vi "Vision Processing.vi"(4 "error in (no error)":errorcluster, 7 "Image Size":T1=enum."320x240") -> ()   [LabVIEW 2015]
doc: "This VI runs in parallel to other tasks. It gets images from the camera, processes them for color or shape and uses commands or globals to affect the behavior of other subsystems."
uses:
  <vilib>/Rock Robotics/WPI/Camera/WPI_CameraImageSize.ctl
  Labview/2016 Vision Tracking/Vision Support Code/Camera Types.ctl
  <vilib>/Rock Robotics/WPI/Camera/WPI_CameraWhite Balance Values.ctl
  <vilib>/Rock Robotics/WPI/Camera/WPI_CameraExposure Values.ctl
  <vilib>/Rock Robotics/WPI/Camera/WPI_CameraFrameRate.ctl
  Framework/Robot Global Data.vi
  <vilib>/vision/NI_Vision_Development_Module.lvlib
panel:
  in  "Max Limit %":dbl=0.12 format="%#_13g"
  in  "Min Limit %":dbl=0.12 format="%#_13g"
  in  "Image Size 2":T1=enum."320x240"
  out "ms to process 2":u32
  in  "error in (no error) 2":errorcluster
  out "ms to process":u32
  in  "LED Color":T2={"Hue"={23.67058792990901, 48.923317529462665}, "Sat"={66.78571428571429, 255.0}, "Val"={48.571428571428584, 255.0}} {"Hue" scale=0.0..255.0 scale format="%#_3g"}
  out "Qualified Particles":i32
  in  "Score Threshold":dbl=75.0
  in  "Aspect Fudge Factor":dbl=1.0
  in  "Min Score Threshold":i32=75
  in  "Camera Type":T3=enum."MS HD3000 square"
  in  "Emphasize Limit Tests":bool=TRUE
  out "Masked 2":T4(plugin-control)
  in  "Display Mask":bool=TRUE
  out "Original Image":T4(plugin-control)
  in  "Display Original":bool=TRUE
  out "Sorted Particle Scores":T5(array[cluster]) {"Moment Factor" format="%#_3g"; "Aspect Ratio" format="%#_3g"; "Area to CH" format="%#_3g"; "X" format="%#_3g"; "Y" format="%#_3g"}
  out "Highest Avg Score":dbl
  out "Detected Targets":T6(array[cluster]) {"Normalized Rect"."Numeric 5" format="%#_2g"; "Normalized Rect"."Numeric 3" format="%#_2g"; "Normalized Rect"."Numeric 2" format="%#_2g"; "Normalized Rect"."Numeric" format="%#_2g"}
  out "fps":dbl
  out "Masked":T4(plugin-control)
  # "Density Profile"
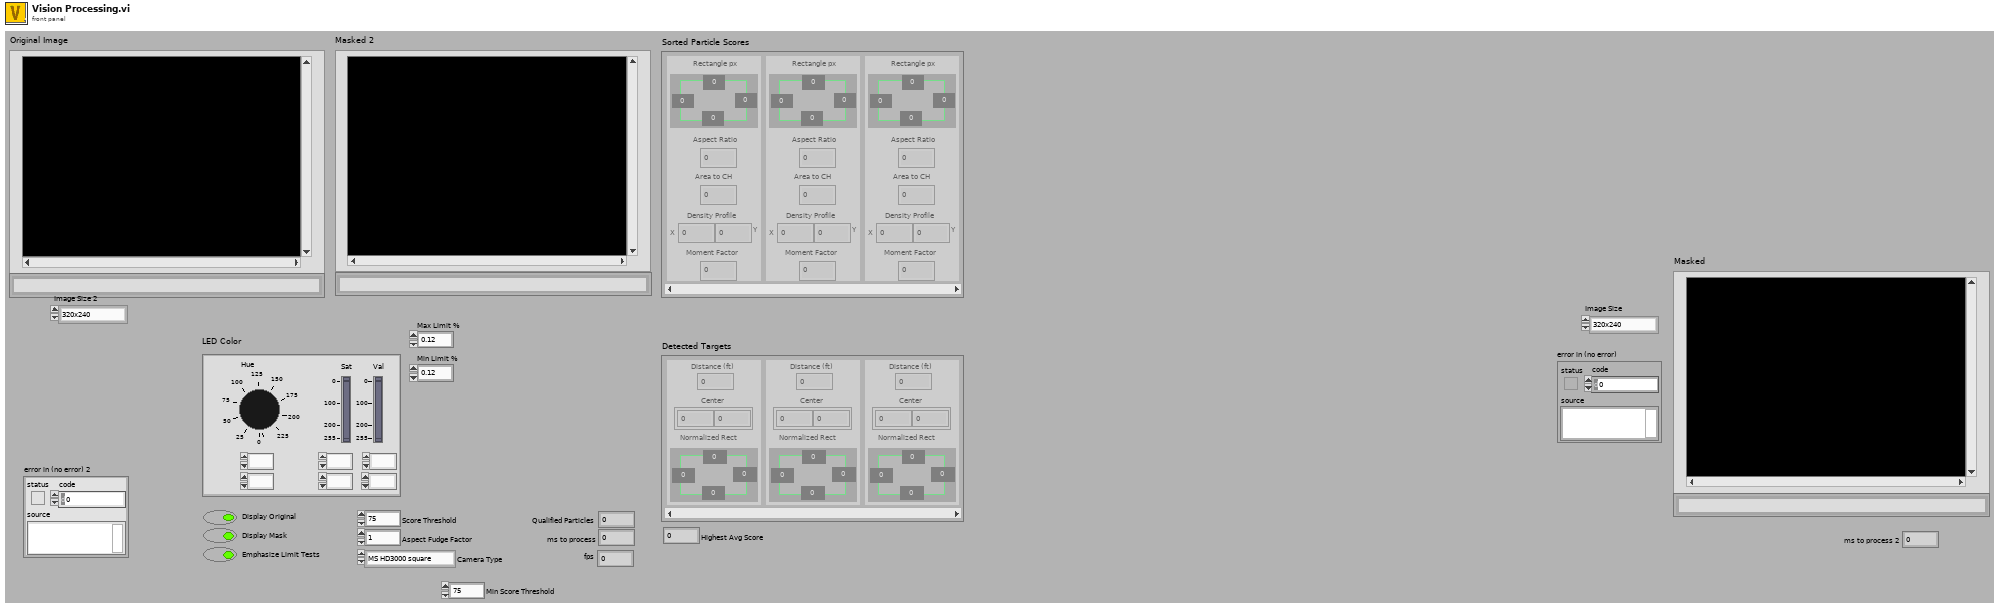
[diagram p1: front panel]
types:
  T1 = typedef "WPI_CameraImageSize.ctl" = enum16{"640x480", "320x240", "160x120", "Custom"}
  T2 = cluster{"Hue":cluster{dbl, dbl}, "Sat":cluster{dbl, dbl}, "Val":cluster{dbl, dbl}}
  T3 = typedef "Camera Types.ctl" = enum16{"206", "1011", "1013", "MS HD3000 square", "MS HD3000 640x480"}
  T4 = typedef "IMAQ Image.ctl" = refnum<image>
  T5 = cluster{"Rectangle px":cluster{"Numeric":dbl, "Numeric 2":dbl, "Numeric 3":dbl, "Numeric 5":dbl}, "Aspect Ratio":dbl, "Area to CH":dbl, "X":dbl, "Y":dbl, "Moment Factor":dbl}[]
  T6 = cluster{"Distance (ft)":dbl, "Center":cluster{dbl, dbl}, "Normalized Rect":cluster{"Numeric":dbl, "Numeric 2":dbl, "Numeric 3":dbl, "Numeric 5":dbl}}[]
  T7 = typedef "WPI_CameraFrameRate.ctl" = u32
  T8 = typedef "WPI_CameraExposure Values.ctl" = enum16{"Auto", "Flicker-free 50 Hz", "Flicker-free 60 Hz", "Hold current", "Custom"}
  T9 = typedef "WPI_CameraWhite Balance Values.ctl" = enum16{"Auto", "Fixed indoor", "Fixed outdoor 1", "Fixed outdoor 2", "Fixed fluorescent 1", "Fixed fluorescent 2", "Hold current", "Custom"}
  T10 = typedef "Image Type" = u32
  T11 = typedef "Particle Parameters" = i32
  T12 = typedef "WPI_CameraDevRef.ctl" = cluster{"Camera Address":string, "CameraStatus":errorcluster}
  T13 = cluster{"Bounding box":cluster{"left":dbl, "top":dbl, "right":dbl, "bottom":dbl}, "Aspect Ratio":dbl, "Area to CH":dbl, "X Mask":dbl, "Y Mask":dbl, "Moment":dbl}[]
  T14 = cluster{"Rectangle":cluster{"Numeric":dbl, "Numeric 2":dbl, "Numeric 3":dbl, "Numeric 5":dbl}, "L":dbl, "Area to CH":dbl, "X":dbl, "Y":dbl, "Moment Factor":dbl}[]
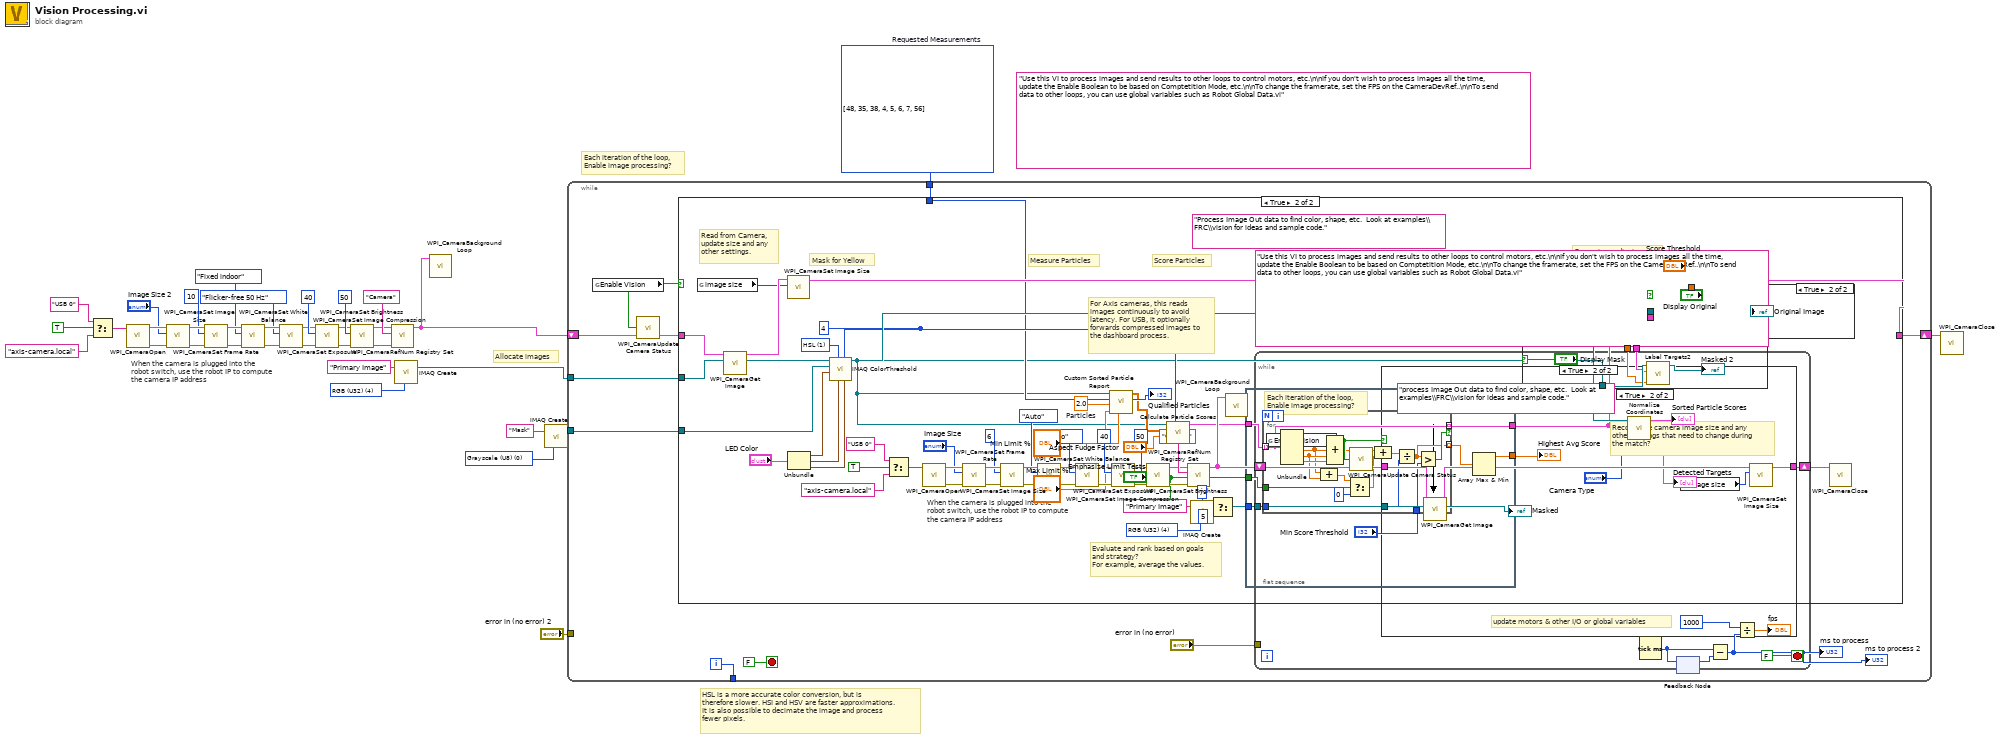
[diagram p0: block diagram]
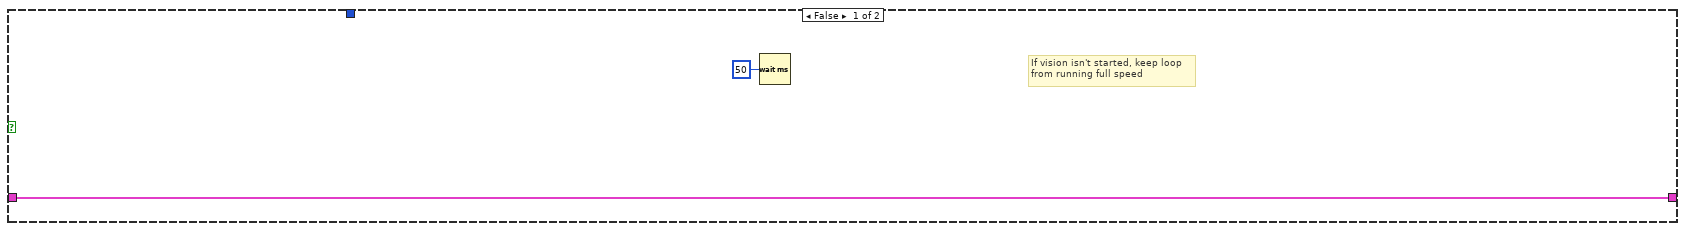
[diagram p2: hidden frame]
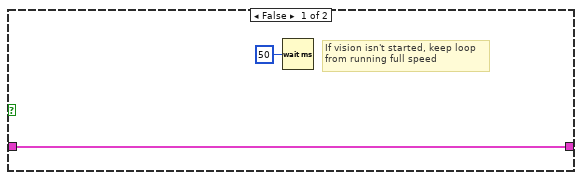
[diagram p5: hidden frame]
diagram:
  w29 = T10 4 items=["Grayscale (U8)", "Grayscale (I16)", "Grayscale (SGL)", "Complex (CSG)", "RGB (U32)", "HSL (U32)", "RGB (U64)"] ("Image Type")
  (unwired) "Use this VI to process images and send results to other loops to control motors, etc.\n\nIf you don't wish to process images all the time, update the Enable Boolean to be based on Comptetition Mode, etc.\n\nTo change the framerate, set the FPS on the CameraDevRef..\n\nTo send data to other loops, you can use global variables such as Robot Global Data.vi"
  w32 = T11[] [48, 35, 38, 4, 5, 6, 7, 56] items=["Center of Mass X", "Center of Mass Y", "First Pixel X", "First Pixel Y", "Bounding Rect Left", "Bounding Rect Top", "Bounding Rect Right", "Bounding Rect Bottom", "Max Feret Diameter Start X", "Max Feret Diameter Start Y", "Max Feret Diameter End X", "Max Feret Diameter End Y", "Max Horiz. Segment Length Left", "Max Horiz. Segment Length Right", "Max Horiz. Segment Length Row", "-", "Bounding Rect Width", "Bounding Rect Height", "Bounding Rect Diagonal", "Perimeter", "Convex Hull Perimeter", "Holes' Perimeter", "Max Feret Diameter", "Equivalent Ellipse Major Axis", "Equivalent Ellipse Minor Axis", "Equivalent Ellipse Minor Axis (Feret)", "Equivalent Rect Long Side", "Equivalent Rect Short Side", "Equivalent Rect Diagonal", "Equivalent Rect Short Side (Feret)", "Average Horiz. Segment Length", "Average Vert. Segment Length", "Hydraulic Radius", "Waddel Disk Diameter", "-", "Area", "Holes' Area", "Particle & Holes' Area", "Convex Hull Area", "Image Area", "-", "Number of Holes", "Number of Horiz. Segments", "Number of Vert. Segments", "-", "Orientation", "Max Feret Diameter Orientation", "-", "% Area/Image Area", "% Area/(Particle & Holes' Area)", "Ratio of Equivalent Ellipse Axes", "Ratio of Equivalent Rect Sides", "-", "Elongation Factor", "Compactness Factor", "Heywood Circularity Factor", "Type Factor", "-", "Sum X", "Sum Y", "Sum XX", "Sum XY", "Sum YY", "Sum XXX", "Sum XXY", "Sum XYY", "Sum YYY", "-", "Moment of Inertia XX", "Moment of Inertia XY", "Moment of Inertia YY", "Moment of Inertia XXX", "Moment of Inertia XXY", "Moment of Inertia XYY", "Moment of Inertia YYY", "Norm. Moment of Inertia XX", "Norm. Moment of Inertia XY", "Norm. Moment of Inertia YY", "Norm. Moment of Inertia XXX", "Norm. Moment of Inertia XXY", "Norm. Moment of Inertia XYY", "Norm. Moment of Inertia YYY", "Hu Moment 1", "Hu Moment 2", "Hu Moment 3", "Hu Moment 4", "Hu Moment 5", "Hu Moment 6", "Hu Moment 7"]  # Requested Measurements
  w35 = T10 0 items=["Grayscale (U8)", "Grayscale (I16)", "Grayscale (SGL)", "Complex (CSG)", "RGB (U32)", "HSL (U32)", "RGB (U64)", "Grayscale (U16)"] ("Image Type")
  (unwired) "Use this VI to process images and send results to other loops to control motors, etc.\n\nIf you don't wish to process images all the time, update the Enable Boolean to be based on Comptetition Mode, etc.\n\nTo change the framerate, set the FPS on the CameraDevRef..\n\nTo send data to other loops, you can use global variables such as Robot Global Data.vi"
  w66 = T10 4 items=["Grayscale (U8)", "Grayscale (I16)", "Grayscale (SGL)", "Complex (CSG)", "RGB (U32)", "HSL (U32)", "RGB (U64)"] ("Image Type")
  # "When the camera is plugged into the\nrobot switch, use the robot IP to compute\nthe camera IP address"
  # "Each iteration of the loop,\nEnable image processing?"
  # "HSL is a more accurate color conversion, but is\ntherefore slower. HSI and HSV are faster approximations.\nIt is also possible to decimate the image and process\nfewer pixels."
  # "Allocate images"
  # "When the camera is plugged into the\nrobot switch, use the robot IP to compute\nthe camera IP address"
  # "For Axis cameras, this reads\nimages continuously to avoid\nlatency. For USB, it optionally\nforwards compressed images to\nthe dashboard process."
  n1 = Select(t="USB 0" ("format string"), s=TRUE ("dot notation? (F)"), f="axis-camera.local" ("format string")) -> (s? t:f=w4:string)
  n2 = call <vilib>:"WPI_CameraOpen.vi"("Camera Address"=w4) -> ("error out"=w18:errorcluster, "CameraDevRef"=w19:T12)  [unwired: 1 in, 8 out]
  n3 = call <vilib>:"WPI_CameraSet Image Size.vi"("error in (no error)"=w18, "Image Size"="Image Size 2", "CameraDevRef"=w19) -> ("error out"=w17:errorcluster, "CameraDevRef Out"=w20:T12)  [unwired: 1 in, 6 out]
  n4 = call <vilib>:"WPI_CameraSet Frame Rate.vi"("error in (no error)"=w17, "Frame Rate (fps)"=T7 10, "CameraDevRef"=w20) -> ("error out"=w16:errorcluster, "CameraDevRef Out"=w22:T12)  [unwired: 7 out]
  n5 = call <vilib>:"WPI_CameraSet White Balance.vi"("error in (no error)"=w16, "White Balance"=WPI_CameraWhite_Balance_Values."Fixed indoor", "CameraDevRef"=w22) -> ("error out"=w15:errorcluster, "CameraDevRef Out"=w21:T12)  [unwired: 1 in, 6 out]
  n6 = call <vilib>:"WPI_CameraSet Exposure.vi"("error in (no error)"=w15, "Exposure"=WPI_CameraExposure_Values."Flicker-free 50 Hz", "CameraDevRef"=w21) -> ("error out"=w14:errorcluster, "CameraDevRef Out"=w24:T12)  [unwired: 1 in, 6 out]
  n7 = call <vilib>:"WPI_CameraSet Image Compression.vi"("error in (no error)"=w14, "Compression"=40, "CameraDevRef"=w24) -> ("error out"=w13:errorcluster, "CameraDevRef Out"=w23:T12)  [unwired: 7 out]
  n8 = call <vilib>:"WPI_CameraSet Brightness.vi"("error in (no error)"=w13, "Brightness"=50, "CameraDevRef"=w23) -> ("error out"=w11:errorcluster, "CameraDevRef Out"=w12:T12)  [unwired: 7 out]
  n9 = call <vilib>:"WPI_CameraRefNum Registry Set.vi"("error in (no error)"=w11, "refnum name"="Camera", "CameraDevRef"=w12) -> ("CameraDevRef"=w2:T12)  [unwired: 1 in, 7 out]
  n10 = call "IMAQ Create"("Image Name"="Primary Image", "Image Type"=w29) -> ("New Image"=w1:T4)  [unwired: 2 in, 2 out]
  n11 = call <vilib>:"WPI_CameraBackground Loop.vi"("CameraDevRef"=w2) -> ()  [unwired: 11 in]
  n12 = call "IMAQ Create"("Image Name"="Mask", "Image Type"=w35) -> ("New Image"=w33:T4)  [unwired: 2 in, 2 out]
  n13 = while {
    tunnel: w1 -> [w75]
    tunnel: w33 -> [w79]
    tunnel: w32 -> [w78]
    tunnel: "error in (no error) 2" -> [_]
    tunnel: [w74] -> _
    shift-right: [w71] -> w30
    shift-left: w2 -> [w67]
    i -> [w74]
    stop <- FALSE stop-if-true
    n14 = global read "Robot Global Data.vi" "Enable Vision"() -> (w73:bool)
    n15 = call <vilib>:"WPI_CameraUpdate Camera Status.vi"("CameraDevRef In"=w67, "Enable Vision"=w73) -> ("CameraDevRef Out"=w72:T12)  [unwired: 3 in]
    n16 = case shown="True" w73 {
      tunnel: w79 -> [_ w116]
      tunnel: w78 -> [_ w87]
      tunnel: w72 -> [w81 w111]
      tunnel: w75 -> [_ w110]
      tunnel: [w81 w108] -> w71
      frame False {
        # "If vision isn't started, keep loop\nfrom running full speed"
        n17 = Wait (ms)(milliseconds to wait=u32 50) -> ()  [unwired: 1 out]
      }
      frame True {
        w95 = 4 ("Replace Value")
        w105 = u16 1 items=["RGB", "HSL", "HSV", "HSI"] ("Color Mode")
        (unwired) "Process Image Out data to find color, shape, etc.  Look at examples\\FRC\\vision for ideas and sample code."
        w85 = 2.0  # Particles
        # "Evaluate and rank based on goals\nand strategy?\nFor example, average the values."
        # "Read from Camera,\nupdate size and any\nother settings."
        # "Measure Particles"
        # "Convert coordinates,\ncalculate distance, etc."
        # "Annotation"
        # "Score Particles"
        # "Mask for Yellow"
        n18 = global read "Robot Global Data.vi" "image size"() -> (w92:T1)
        n19 = call <vilib>:"WPI_CameraGet Image.vi"("Image"=w110, "CameraDevRef"=w111) -> ("Image Out"=w96:T4, "CameraDevRef Out"=w109:T12)  [unwired: 7 in, 1 out]
        n20 = call <vilib>:"WPI_CameraSet Image Size.vi"("Image Size"=w92, "CameraDevRef"=w109) -> ("CameraDevRef Out"=w108:T12)  [unwired: 2 in, 7 out]
        n21 = Unbundle("LED Color") -> ("Hue"=w115:cluster{dbl, dbl}, "Sat"=w114:cluster{dbl, dbl}, "Val"=w113:cluster{dbl, dbl})
        n22 = call "IMAQ ColorThreshold"("Blue or Luma or Val or Inten Range"=w113, "Replace Value"=w95, "Green or Sat Range"=w114, "Color Mode"=w105, "Red or Hue Range"=w115, "Image Dst"=w116, "Image Src"=w96) -> ("Image Dst Out"=w83:T4)  [unwired: 3 in, 1 out]
        n23 = call "Custom Sorted Particle Report.vi"("Min Area Size %"="Min Limit %", "Max Area Size %"="Max Limit %", "Particle Count Limit"=w85, "Pixel Measurements"=w87, "Image in"=w83) -> ("Particles"=→"Qualified Particles":i32, "Sorted Data"=w88:dbl[][])  [unwired: 5 in]
        n24 = call "Calculate Particle Scores.vi"("Pixel Value"=w95, "Aspect Fudge Factor"="Aspect Fudge Factor", "Sorted Data"=w88, "Image in"=w83) -> ("Scores"=w103:T13)  [unwired: 7 in]
        n25 = Select(t=7, s="Emphasize Limit Tests", f=5) -> (s? t:f=w100:i32)
        n26 = flat-sequence {
          tunnel: w103 -> [w127]
          tunnel: w100 -> [w125]
          tunnel: [w128] -> w99
          tunnel: [w122] -> w91
          tunnel: "Emphasize Limit Tests" -> [w126]
          frame #0 {
            n27 = for {
              tunnel: w127 -> [w142] mode=indexing
              tunnel: [w142] -> w122 mode=indexing if=w141
              tunnel: [w140] -> w123 mode=indexing
              tunnel: w125 -> [w139]
              tunnel: "Min Score Threshold" -> [w138]
              tunnel: w126 -> [w131]
              n28 = Unbundle(w142) -> ("Aspect Ratio"=w144:dbl, "Area to CH"=w143:dbl, "X Mask"=w133:dbl, "Y Mask"=w134:dbl, "Moment"=w135:dbl)  [unwired: 1 out]
              n29 = Compound Arithmetic op=ADD(w133, w134) -> (w132:dbl)
              n30 = Compound Arithmetic op=ADD(w144, w143, w133, w134, w135) -> (w137:dbl)
              n31 = Select(t=w132, s=w131, f=0) -> (s? t:f=w130:dbl)
              n32 = Compound Arithmetic op=ADD(w137, w130) -> (w136:dbl)
              n33 = Divide(x=w136, y=w139) -> (x/y=w140:dbl)
              n34 = Greater?(x=w140, y=w138) -> (0:w141:bool)
            }
            n35 = Array Max & Min(array=w123) -> (max value=w128:dbl)  [unwired: 3 out]
          }
        }
        n36 = case shown="True" "Display Mask" {
          tunnel: w83 -> [_ w121]
          tunnel: w91 -> [_ w119]
          tunnel: "Score Threshold" -> [_ w118]
          frame False {
          }
          frame True {
            n37 = call "Label Targets2.vi"("Score Threshold"=w118, "Targets"=w119, "Image in"=w121) -> ("Image out"=→"Masked 2":T4)  [unwired: 8 in]
          }
        }
        n38 = call "Normalize Coordinates.vi"("Camera Type"="Camera Type", "Targets"=w91, "Image in"=w96) -> ("Found Targets"=→"Detected Targets":T6, "Sorted Scores"=→"Sorted Particle Scores":T14)  [unwired: 7 in]
        n39 = case shown="True" "Display Original" {
          tunnel: w96 -> [_ w117]
          tunnel: w91 -> [_ _]
          tunnel: "Score Threshold" -> [_ _]
          frame False {
          }
          frame True {
            "Original Image" <- w117
          }
        }
        "Highest Avg Score" <- w99
      }
    }
    n40 = Tick Count (ms)() -> (millisecond timer value=w76:u32)
    n41 = feedback-in #1(w76) -> ()
    n42 = feedback #1() -> (w77:u32)  [unwired: 1 in]
    n43 = Subtract(x=w76, y=w77) -> (x-y=w68:u32)
    "ms to process" <- w68
    "ms to process 2" <- w68
    n44 = Divide(x=1000 ("Brightness"), y=w68) -> (x/y=→"fps":dbl)
  }
  n45 = Select(t="USB 0" ("format string"), s=TRUE ("dot notation? (F)"), f="axis-camera.local" ("format string")) -> (s? t:f=w37:string)
  n46 = call <vilib>:"WPI_CameraOpen.vi"("Camera Address"=w37) -> ("error out"=w54:errorcluster, "CameraDevRef"=w55:T12)  [unwired: 1 in, 8 out]
  n47 = call <vilib>:"WPI_CameraSet Image Size.vi"("error in (no error)"=w54, "Image Size"="Image Size", "CameraDevRef"=w55) -> ("error out"=w53:errorcluster, "CameraDevRef Out"=w56:T12)  [unwired: 1 in, 6 out]
  n48 = call <vilib>:"WPI_CameraSet Frame Rate.vi"("error in (no error)"=w53, "Frame Rate (fps)"=T7 6, "CameraDevRef"=w56) -> ("error out"=w52:errorcluster, "CameraDevRef Out"=w58:T12)  [unwired: 7 out]
  n49 = call <vilib>:"WPI_CameraSet White Balance.vi"("error in (no error)"=w52, "White Balance"=WPI_CameraWhite_Balance_Values."Auto", "CameraDevRef"=w58) -> ("error out"=w51:errorcluster, "CameraDevRef Out"=w57:T12)  [unwired: 1 in, 6 out]
  n50 = call <vilib>:"WPI_CameraSet Exposure.vi"("error in (no error)"=w51, "Exposure"=WPI_CameraExposure_Values."Auto", "CameraDevRef"=w57) -> ("error out"=w50:errorcluster, "CameraDevRef Out"=w60:T12)  [unwired: 1 in, 6 out]
  n51 = call <vilib>:"WPI_CameraSet Image Compression.vi"("error in (no error)"=w50, "Compression"=40, "CameraDevRef"=w60) -> ("error out"=w49:errorcluster, "CameraDevRef Out"=w59:T12)  [unwired: 7 out]
  n52 = call <vilib>:"WPI_CameraSet Brightness.vi"("error in (no error)"=w49, "Brightness"=50, "CameraDevRef"=w59) -> ("error out"=w47:errorcluster, "CameraDevRef Out"=w48:T12)  [unwired: 7 out]
  n53 = call <vilib>:"WPI_CameraRefNum Registry Set.vi"("error in (no error)"=w47, "refnum name"="Camera", "CameraDevRef"=w48) -> ("CameraDevRef"=w43:T12)  [unwired: 1 in, 7 out]
  n54 = call "IMAQ Create"("Image Name"="Primary Image", "Image Type"=w66) -> ("New Image"=w64:T4)  [unwired: 2 in, 2 out]
  n55 = call <vilib>:"WPI_CameraBackground Loop.vi"("CameraDevRef"=w43) -> ()  [unwired: 11 in]
  n56 = while {
    shift-right: [w149] -> w41
    shift-left: w43 -> [w147]
    tunnel: w64 -> [w148]
    tunnel: "error in (no error)" -> [_]
    stop <- FALSE stop-if-true
    # "Each iteration of the loop,\nEnable image processing?"
    n57 = global read "Robot Global Data.vi" "Enable Vision"() -> (w145:bool)
    n58 = call <vilib>:"WPI_CameraUpdate Camera Status.vi"("CameraDevRef In"=w147, "Enable Vision"=w145) -> ("CameraDevRef Out"=w146:T12)  [unwired: 3 in]
    n59 = case shown="True" w145 {
      tunnel: w148 -> [_ w157]
      tunnel: [w152 w158] -> w149
      tunnel: w146 -> [w152 w155]
      frame False {
        # "If vision isn't started, keep loop\nfrom running full speed"
        n60 = Wait (ms)(milliseconds to wait=u32 50) -> ()  [unwired: 1 out]
      }
      frame True {
        (unwired) "process Image Out data to find color, shape, etc.  Look at examples\\FRC\\vision for ideas and sample code."
        # "update motors & other I/O or global variables"
        # "Reconfigure camera image size and any\nother settings that need to change during\nthe match?"
        n61 = call <vilib>:"WPI_CameraGet Image.vi"("Image"=w157, "CameraDevRef"=w155) -> ("Image Out"=→"Masked":T4, "CameraDevRef Out"=w154:T12)  [unwired: 1 in, 7 out]
        n62 = global read "Robot Global Data.vi" "image size"() -> (w156:T1)
        n63 = call <vilib>:"WPI_CameraSet Image Size.vi"("Image Size"=w156, "CameraDevRef"=w154) -> ("CameraDevRef Out"=w158:T12)  [unwired: 2 in, 7 out]
      }
    }
  }
  n64 = call <vilib>:"WPI_CameraClose.vi"("CameraDevRef"=w41) -> ()  [unwired: 1 in, 10 out]
  n65 = call <vilib>:"WPI_CameraClose.vi"("CameraDevRef"=w30) -> ()  [unwired: 1 in, 10 out]
